vi "Close PolarizationProcessor.vi"(8 "error in (no error)":errorcluster, 11 "PolarizationProcessor reference":refnum<k24>) -> (0 "error out":errorcluster)   [LabVIEW 2015]
uses:
  C:/code/Host/Installer/Scientific Camera Interfaces/LabVIEW/64_bit/Library_X64/Thorlabs.TSI.PolarizationInterfaces.dll
  64_bit/Library_X64/Thorlabs.TSI.PolarizationInterfaces.dll
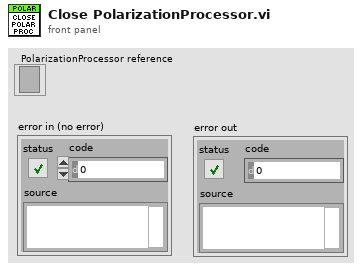
[diagram p1: front panel]
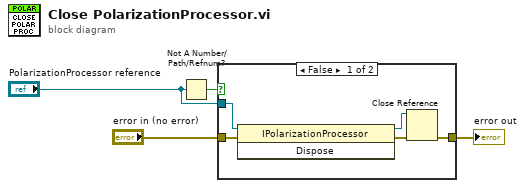
[diagram p0: block diagram]
diagram:
  n1 = Not A Number/Path/Refnum?(number/path/refnum="PolarizationProcessor reference") -> (NaN/Path/Refnum?=w2:bool)
  n2 = case shown="False" w2 {
    tunnel: [w7 w10] -> w4
    tunnel: "error in (no error)" -> [w6 w10]
    tunnel: "PolarizationProcessor reference" -> [w5 _]
    frame False {
      n3 = invoke class="IPolarizationProcessor" method="Dispose"(reference=w5, error in=w6) -> (reference out=w8:refnum<k24>, error out=w9:errorcluster)  [unwired: 1 in, 1 out]
      n4 = Close Reference(reference=w8, error in (no error)=w9) -> (error out=w7:errorcluster)
    }
    frame True {
    }
  }
  "error out" <- w4
